vi "Select email recipient from list.vi"(8 "error in (no error)":errorcluster, 11 "Path":path) -> (0 "error out":errorcluster, 3 "String":string)   [LabVIEW 2013]
panel:
  in  "done":bool
  in  "Email recipients (press control for multiple items)":i32[](listbox)
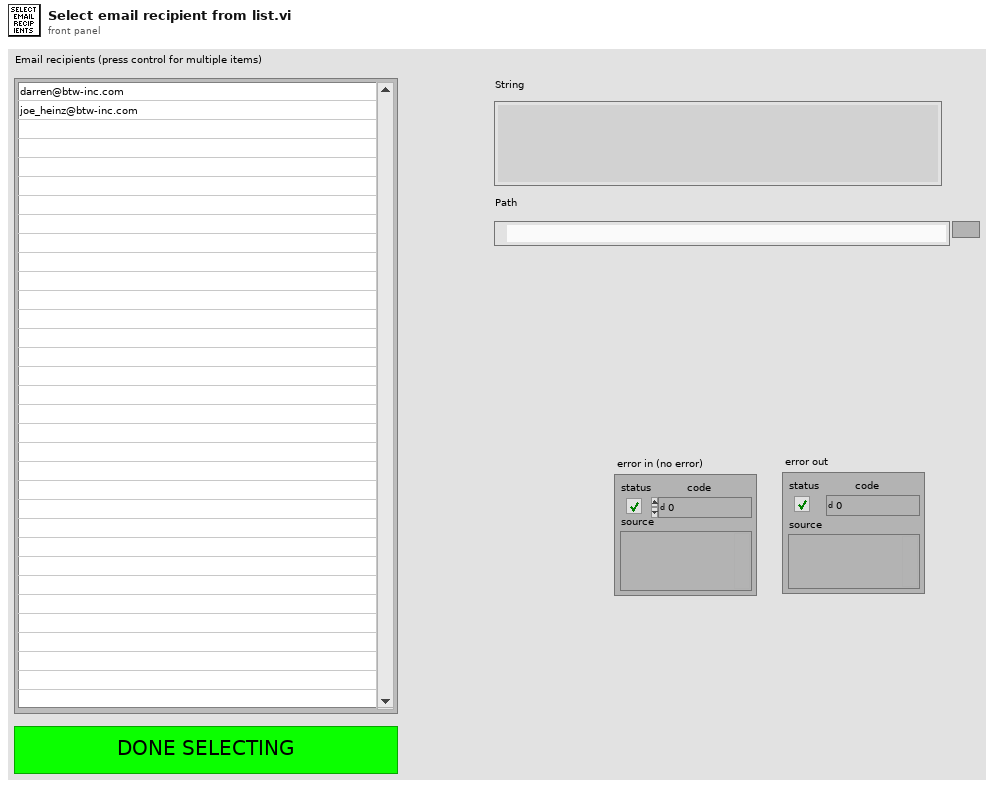
[diagram p1: front panel]
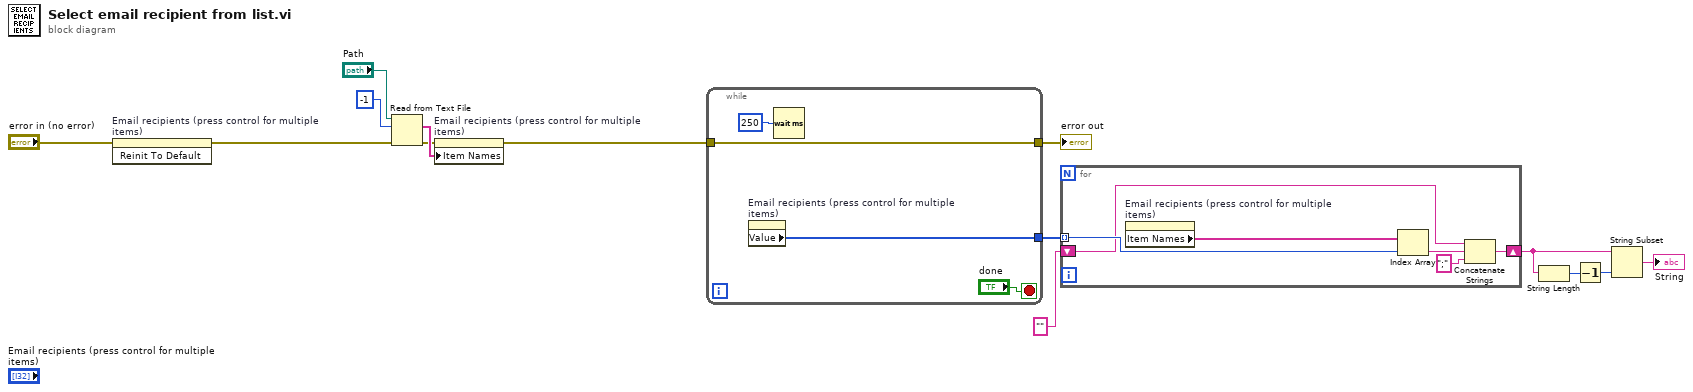
[diagram p0: block diagram]
diagram:
  n1 = invoke on="Email recipients (press control for multiple items)" class="LstBox (strict)" method="Reinit To Default"(error in="error in (no error)") -> (error out=w1:errorcluster)  [unwired: 2 in, 2 out]
  n2 = Read from Text File(file (use dialog)="Path", count=-1, error in=w1) -> (text=w10:string[], error out=w9:errorcluster)  [unwired: 1 in, 2 out]
  n3 = property on="Email recipients (press control for multiple items)" class="LstBox (strict)"(error in=w9, "Item Names"=w10) -> (error out=w3:errorcluster)  [unwired: 1 in, 1 out]
  n4 = while {
    tunnel: [w17] -> w13
    tunnel: w3 -> [w16]
    tunnel: [w16] -> w8
    stop <- "done" stop-if-true
    n5 = property on="Email recipients (press control for multiple items)" class="LstBox (strict)"() -> ("Value"=w17:i32[])  [unwired: 2 in, 2 out]
    n6 = Wait (ms)(milliseconds to wait=u32 250) -> ()  [unwired: 1 out]
  }
  "error out" <- w8
  n7 = for {
    tunnel: w13 -> [w23] mode=indexing
    shift-right: [w19] -> w7
    shift-left: "" -> [w22]
    n8 = property on="Email recipients (press control for multiple items)" class="LstBox (strict)"() -> ("Item Names"=w24:string[])  [unwired: 2 in, 2 out]
    n9 = Index Array(array=w24, index=w23) -> (element=w21:string)
    n10 = Concatenate Strings(w22, w21, ";" ("string")) -> (w19:string)
  }
  n11 = String Length(string=w7) -> (length=w6:i32)
  n12 = Decrement(x=w6) -> (x-1=w5:i32)
  n13 = String Subset(string=w7, length (rest)=w5) -> (substring=→"String":string)  [unwired: 1 in]
